vi "Load_Zspec_param_data_SubVI.vi"(10 "data\n\n 5":T1(array[cluster]), 11 "Zspecparam.txt location":path) -> (3 "data":T1(array[cluster]))   [LabVIEW 2014]
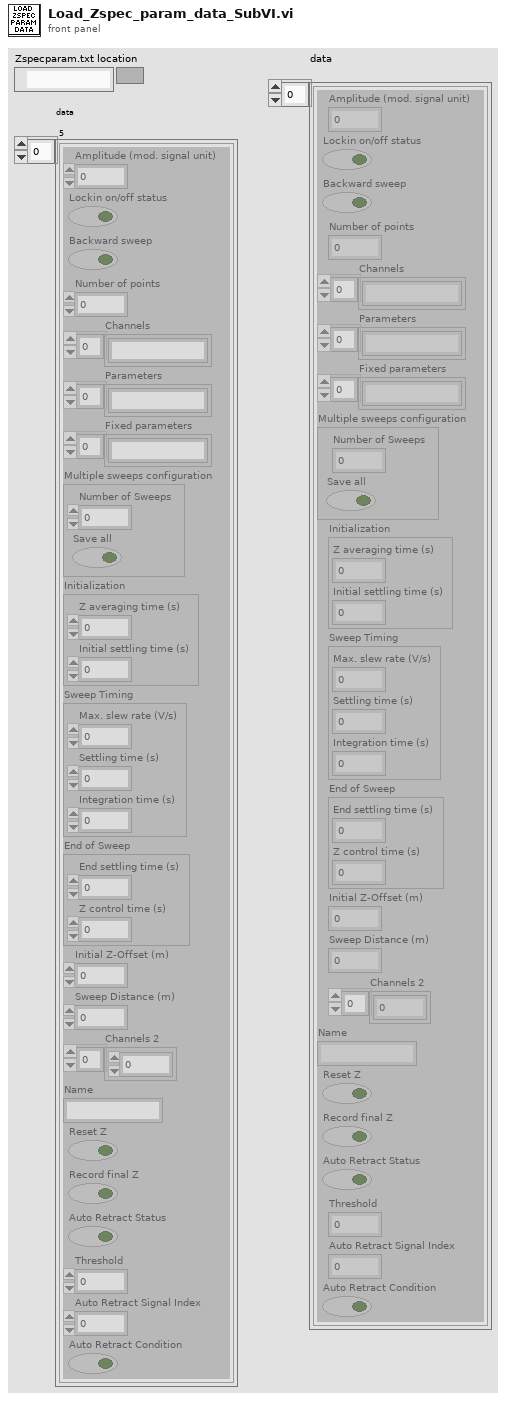
[diagram p1: front panel]
types:
  T1 = cluster{"Amplitude (mod. signal unit)":sgl, "Lockin on/off status":bool, "Backward sweep":bool, "Number of points":i32, "Channels":string[], "Parameters":string[], "Fixed parameters":string[], "Multiple sweeps configuration":cluster{"Number of Sweeps":i32, "Save all":bool}, "Initialization":cluster{"Z averaging time (s)":sgl, "Initial settling time (s)":sgl}, "Sweep Timing":cluster{"Max. slew rate (V/s)":sgl, "Settling time (s)":sgl, "Integration time (s)":sgl}, "End of Sweep":cluster{"End settling time (s)":sgl, "Z control time (s)":sgl}, "Initial Z-Offset (m)":sgl, "Sweep Distance (m)":sgl, "Channels 2":i32[], "Name":string, "Reset Z":bool, "Record final Z":bool, "Auto Retract Status":bool, "Threshold":sgl, "Auto Retract Signal Index":i32, "Auto Retract Condition":bool}[]
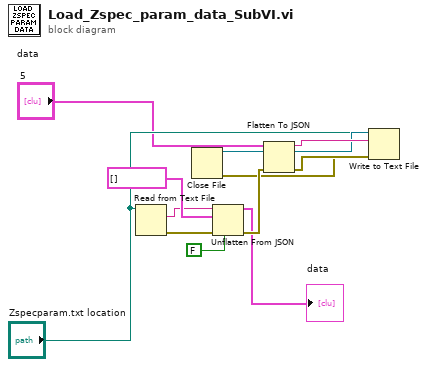
[diagram p0: block diagram]
diagram:
  n1 = Read from Text File(file (use dialog)="Zspecparam.txt location") -> (text=w1:string, error out=w12:errorcluster)  [unwired: 3 in, 2 out]
  n2 = Unflatten From JSON(JSON string=w1, type and defaults=T1 [] ("data"), default null elements? (F)=FALSE, error in (no error)=w12) -> (value=→"data":T1, error out=w11:errorcluster)  [unwired: 3 in]
  n3 = Flatten To JSON(anything="data\n\n 5", error in (no error)=w11) -> (JSON string=w9:string, 11:w10:errorcluster)  [unwired: 1 in]
  n4 = Write to Text File(file (use dialog)="Zspecparam.txt location", text=w9, error in=w10) -> (refnum out=w7:refnum<file>, error out=w8:errorcluster)  [unwired: 1 in, 1 out]
  n5 = Close File(refnum=w7, error in=w8) -> ()  [unwired: 2 out]
